vi "types_of_arrays.vi"() -> ()   [LabVIEW 2019]
panel:
  out "4D":dbl[][][][](array[numeric])
  in  "4 Dimentional array":dbl[][][][](array[numeric])
  out "3D":dbl[][][](array[numeric])
  in  "3 Dimentional array":dbl[][][](array[numeric])
  out "2D":dbl[][](array[numeric])
  in  "2 Dimentional array":dbl[][](array[numeric])
  out "1D":dbl[](array[numeric])
  in  "1Dimentional array":dbl[](array[numeric])
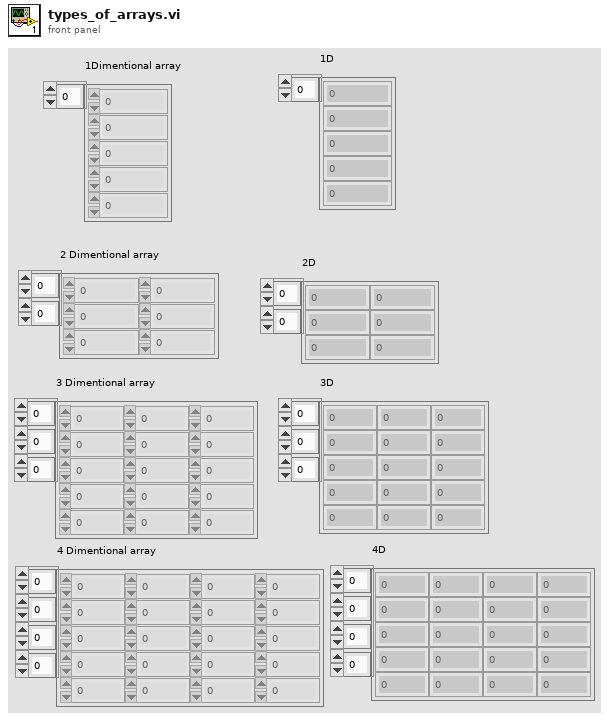
[diagram p1: front panel]
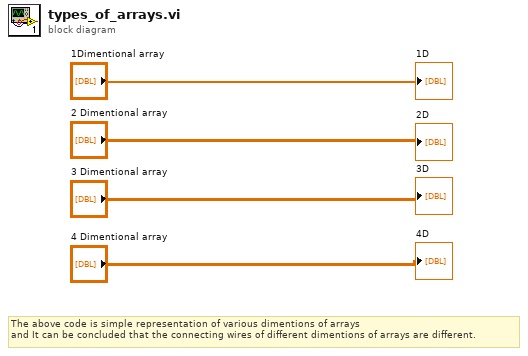
[diagram p0: block diagram]
diagram:
  # "The above code is simple representation of various dimentions of arrays\nand It can be concluded that the connecting wires of different dimentions of arrays are different."
  "1D" <- "1Dimentional array"
  "2D" <- "2 Dimentional array"
  "3D" <- "3 Dimentional array"
  "4D" <- "4 Dimentional array"
